vi "Get AccessType+.vi"(8 "Error In":errorcluster, 11 "reference in":refnum<class "OD Entry.lvclass">) -> (0 "Error Out":errorcluster, 1 "Defined?":bool, 2 "AccessType":T1=enum."const", 3 "reference out":refnum<class "OD Entry.lvclass">)   [LabVIEW 2024, in "EDS.lvlib" / "OD Entry.lvclass"]
uses:
  OD Entry.lvclass
  OD Entry.lvclass/OD Entry.ctl
  Object Type/Object Type Base.lvclass
  Access Type.ctl
  EDS.lvlib
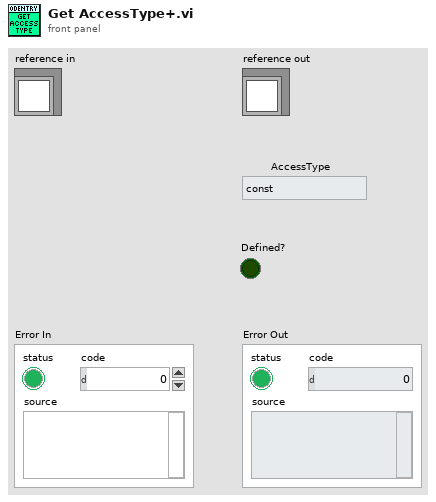
[diagram p1: front panel]
types:
  T1 = typedef "EDS.lvlib/Access Type.ctl" = enum16{"ro", "wo", "rw", "rwr", "rww", "const"}
  T2 = typedef "EDS.lvlib/OD Entry.lvclass/ObjectAttributes.ctl" = cluster{"Index":u16, "ObjectType":refnum<class "Object Type Base.lvclass">, "Denotation":string, "Count":u8, "ObjExtend":u8, "PDOtype":T3, "Label":string, "Description":string, "Sub-Entries":map{u16, refnum<class "OD Sub-Entry.lvclass">}}
  T3 = typedef "EDS.lvlib/PDO Mapping Type.ctl" = enum16{"NO", "OPTIONAL", "RPDO", "TPDO", "DEFAULT"}
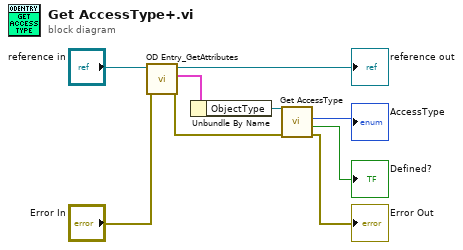
[diagram p0: block diagram]
diagram:
  n1 = call "OD Entry_GetAttributes.vi"("Error In"="Error In", "reference in"="reference in") -> ("Error Out"=w3:errorcluster, "Data"=w5:T2, "reference out"=→"reference out":refnum<class "OD Entry.lvclass">)  [unwired: 6 in, 1 out]
  n2 = Unbundle By Name(w5) -> ("ObjectType"=w4:refnum<class "Object Type Base.lvclass">)
  n3 = call-dynamic "Get AccessType.vi"("error in"=w3, "Object Type in"=w4) -> ("error out"=→"Error Out":errorcluster, "Defined?"=→"Defined?":bool, "AccessType"=→"AccessType":T1)  [unwired: 6 in, 1 out]
